vi "Configure Network Adapter.vi"(8 "error in (no error)":errorcluster, 10 "Network Adapter (\"\")":string, 11 "VISA resource name":refnum<visa-resource-name>) -> (0 "error out":errorcluster, 3 "VISA resource name out":refnum<visa-resource-name>)   [LabVIEW 2020, in "Rohde&Schwarz CMXP Base.lvlib"]
doc: "Selects a LAN network adapter for configuration via other SYSTem:COMMunicate:NET:... commands.\n\nAttribute:\nRSCMXPBASE_ATTR_CONFIGURE_NETWORK_ADAPTER\n\nRemote-control command:\nSYSTem:COMMunicate:NET:ADAPter"
uses:
  <instrlib>/Rohde&Schwarz CMXP Base/Rohde&Schwarz CMXP Base.lvlib
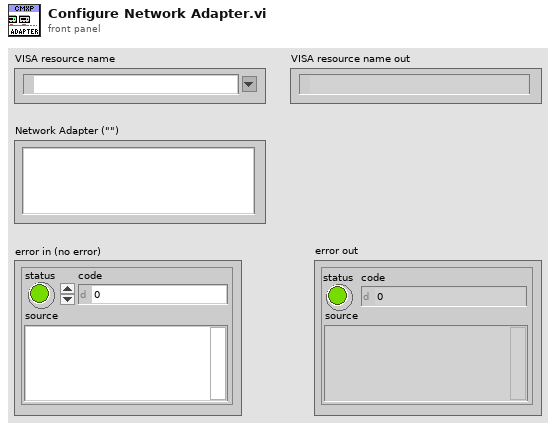
[diagram p1: front panel]
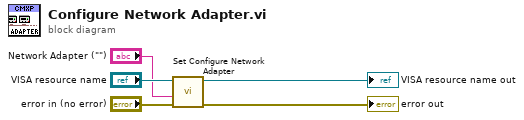
[diagram p0: block diagram]
diagram:
  n1 = call "Set Configure Network Adapter"("error in (no error)"="error in (no error)", "Configure Network Adapter ()"="Network Adapter (\"\")", "instrument handle"="VISA resource name") -> ("error out"=→"error out":errorcluster, "instrument handle out"=→"VISA resource name out":refnum<visa-resource-name>)  [unwired: 7 in]
